vi "set_timeouts.vi"(1 "read_timeout (ms); def=1000":i32=1000, 2 "write_timeout (ms); def=1000":i32=1000, 5 "error in (no error)":errorcluster) -> (19 "error out":errorcluster)   [LabVIEW 2020, in "classes.lvlib" / "_Controller.lvclass"]
doc: "Sets both USB read and write timeouts (in milliseconds). Applies to all attached devices.\n\nImplementss the USB Communication API function \"fnPerformaxComSetTimeouts\". \n\nProduced By:\n\n<B>Kod Integrations, LLC</B>\n4835 Marianne Drive\nMount Airy, MD 21771\nhttp://www.kodintegrations.com\nemail: info@kodintegrations.com\nphone: (240) 687-1288"
uses:
  _Controller.lvclass
  error_actions.ctl
  PerformaxCom.dll
  common.lvlib
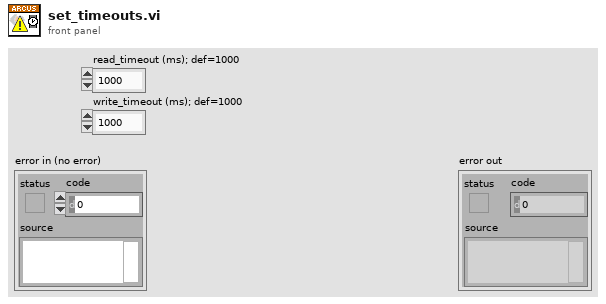
[diagram p1: front panel]
types:
  T1 = typedef "common.lvlib/error_actions.ctl" = enum16{"clearBuff", "closeRef", "nodeErr", "noDeviceInfo", "noDevices", "openRef", "sendReceive", "setTimeouts", "unknown"}
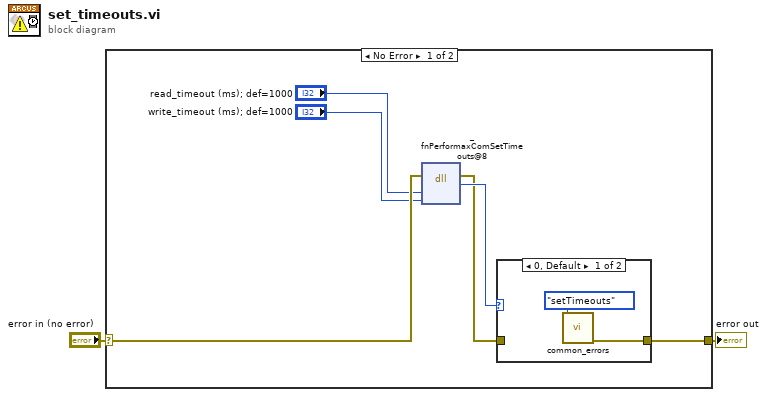
[diagram p0: block diagram]
diagram:
  n1 = case shown="No Error" "error in (no error)" {
    selector: "error in (no error)" -> [w6 w12]
    tunnel: [w5 w12] -> w1
    frame No Error {
      n2 = dll-call lib="PerformaxCom.dll" fn="_fnPerformaxComSetTimeouts@8"(error in=w6, "readTimeout"="read_timeout (ms); def=1000", "writeTimeout"="write_timeout (ms); def=1000") -> (error out=w7:errorcluster, w8:i32)  [unwired: 4 in, 1 out]
      n3 = case shown="0, Default" w8 {
        tunnel: [w9 w11] -> w5
        tunnel: w7 -> [_ w11]
        frame 0, Default {
          n4 = call "common_errors.vi"("common_errors"=error_actions."setTimeouts" ("errors")) -> ("error out"=w9:errorcluster)  [unwired: 14 in]
        }
        frame 1 {
        }
      }
    }
    frame Error {
    }
  }
  "error out" <- w1
